vi "Get Version.vi"(8 "error in (no error)":errorcluster, 11 "VISA resource name":refnum<visa-resource-name>) -> (0 "error out":errorcluster, 2 "Version":string, 3 "VISA resource name out":refnum<visa-resource-name>)   [LabVIEW 2022 SP3, in "Keithley 2450.lvlib"]
doc: "This gets the Present SCPI Version"
uses:
  Keithley 2450.lvlib
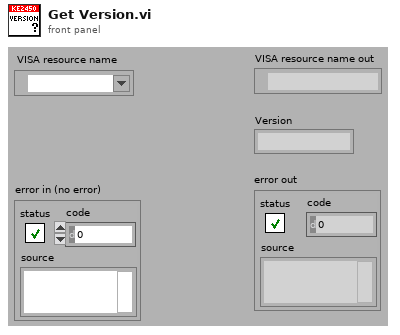
[diagram p1: front panel]
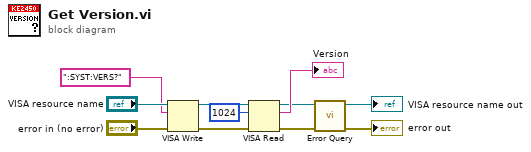
[diagram p0: block diagram]
diagram:
  n1 = VISA Write(VISA resource name="VISA resource name", write buffer=":SYST:VERS?", error in (no error)="error in (no error)") -> (VISA resource name out=w10:refnum<visa-resource-name>, error out=w11:errorcluster)  [unwired: 1 out]
  n2 = VISA Read(VISA resource name=w10, byte count=u32 1024, error in (no error)=w11) -> (VISA resource name out=w3:refnum<visa-resource-name>, read buffer=→"Version":string, error out=w2:errorcluster)  [unwired: 1 out]
  n3 = call "Error Query.vi"("error in (no error)"=w2, "VISA resource name"=w3) -> ("error out"=→"error out":errorcluster, "VISA resource name out"=→"VISA resource name out":refnum<visa-resource-name>)  [unwired: 8 out]
